vi "String to Tree.VI"(2 "error in (no error)":errorcluster, 3 "user formula":string) -> (0 "error out":errorcluster, 1 "Tree formula":T1(array[cluster]))   [LabVIEW 2009]
panel:
  out "error in formula":string
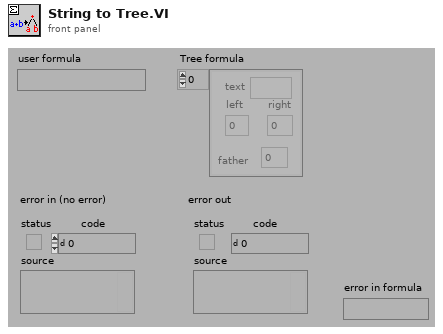
[diagram p1: front panel]
types:
  T1 = cluster{"text":string, "left":i32, "right":i32, "father":i32}[]
  T2 = cluster{"text":string, "left":i32, "right":i32, "father":i32}
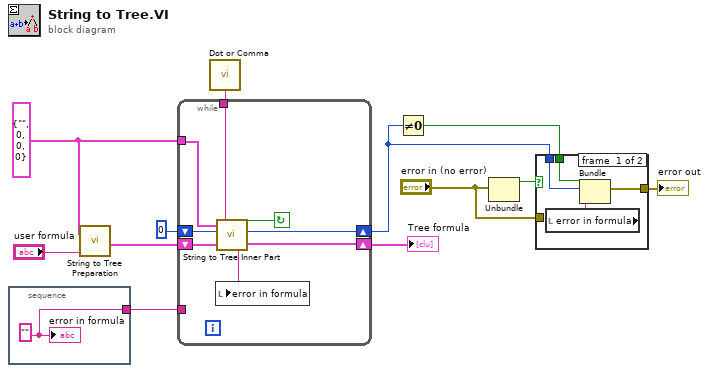
[diagram p0: block diagram]
diagram:
  w1 = T2 {"text"="", "left"=0, "right"=0, "father"=0} ("dummy")
  n1 = stacked-sequence {
    tunnel: [w13] -> w4
    frame #0 {
      w13 = ""
      "error in formula" <- w13
    }
  }
  n2 = call "String to Tree Preparation.vi"("user formula"="user formula", "dummy"=w1) -> ("empty structure"=w12:T1)
  n3 = call "Dot or Comma.vi"() -> ("dot or comma"=w3:string)
  n4 = while {
    tunnel: w3 -> [w16]
    tunnel: w4 -> [_]
    shift-left: 0 -> [w18]
    shift-right: [w19] -> w6
    tunnel: w1 -> [w21]
    shift-left: w12 -> [w20]
    shift-right: [w15] -> w2
    stop <- w17 continue-if-true
    n5 = call "String to Tree Inner Part.vi"("structure before"=w20, "dummy"=w21, "error situation before"=w18, "dot or comma"=w16) -> ("error in formula-write"=w14:string, "structure after"=w15:T1, "error situation after"=w19:i32, "end of analysis"=w17:bool)
    n6 = local write "error in formula"(w14) -> ()
  }
  "Tree formula" <- w2
  n7 = Not Equal To 0?(x=w6) -> (x != 0?=w5:bool)
  n8 = Unbundle("error in (no error)") -> ("status"=w9:bool)  [unwired: 2 out]
  n9 = case shown="False" w9 {
    tunnel: "error in (no error)" -> [_ w26]
    tunnel: [w25 w26] -> w7
    tunnel: w6 -> [w24 _]
    tunnel: w5 -> [w23 _]
    frame #0 {
      n10 = local read "error in formula"() -> (w22:string)
      n11 = Bundle(w23, w24, "error in formula"=w22) -> (w25:cluster{bool, i32, "error in formula":string})  [unwired: 1 in]
    }
    frame #1 {
    }
  }
  "error out" <- w7
